vi "BallPlacementEnemyTactic.vi"(8 "error in (no error)":errorcluster, 9 "Robot":refnum<class "Robot.lvclass">, 10 "Game":refnum<class "Game.lvclass">, 11 "BallPlacementEnemyTactic in":refnum<class "BallPlacementEnemyTactic.lvclass">) -> (0 "error out":errorcluster, 2 "Robot out":refnum<class "Robot.lvclass">, 3 "BallPlacementEnemyTactic out":refnum<class "BallPlacementEnemyTactic.lvclass">)   [LabVIEW 2020, in "BallPlacementEnemyTactic.lvclass"]
uses:
  BallPlacementEnemyTactic.lvclass
  Robot_class/Robot.lvclass
  Game_class/Game.lvclass
  Robot_class/tactics.ctl
  Tactic_class/Tactic.lvclass/Tactic.ctl
  Object_class/Object.lvclass/Object.ctl
  Game_class/Game.lvclass/Game.ctl
  Skillbook_class/Skillbook.lvclass/Skillbook.ctl
  Robot_class/Robot.lvclass/Robot.ctl
  <vilib>/Analysis/baseanly.llb/Unit Vector (DBL).vi
  Game_class/Read Referee.vi
  Game_class/Read BallRef.vi
  Object_class/Read x.vi
  Object_class/Read y.vi
  Skillbook_class/Read HaltSkill.vi
  <vilib>/Analysis/coordinate.llb/2D Cartesian Coordinate Rotation (Scalar).vi
  <vilib>/Analysis/baseanly.llb/Real Dot Product.vi
  Robot_class/Write dest_x.vi
  Robot_class/Write dest_y.vi
  Tactic_class/Read Skillbook.vi
  Robot_class/Write tactic.vi
  Ball_class/Ball.lvclass
  Skillbook_class/Skillbook.lvclass
  Referee_class/Referee.lvclass
  HaltSkill_class/HaltSkill.lvclass
  Utilities_class/Utilities.lvclass
  <vilib>/Analysis/NI_AALPro.lvlib
  <vilib>/Analysis/NI_AALBase.lvlib
panel:
  out "x .or. y?":bool
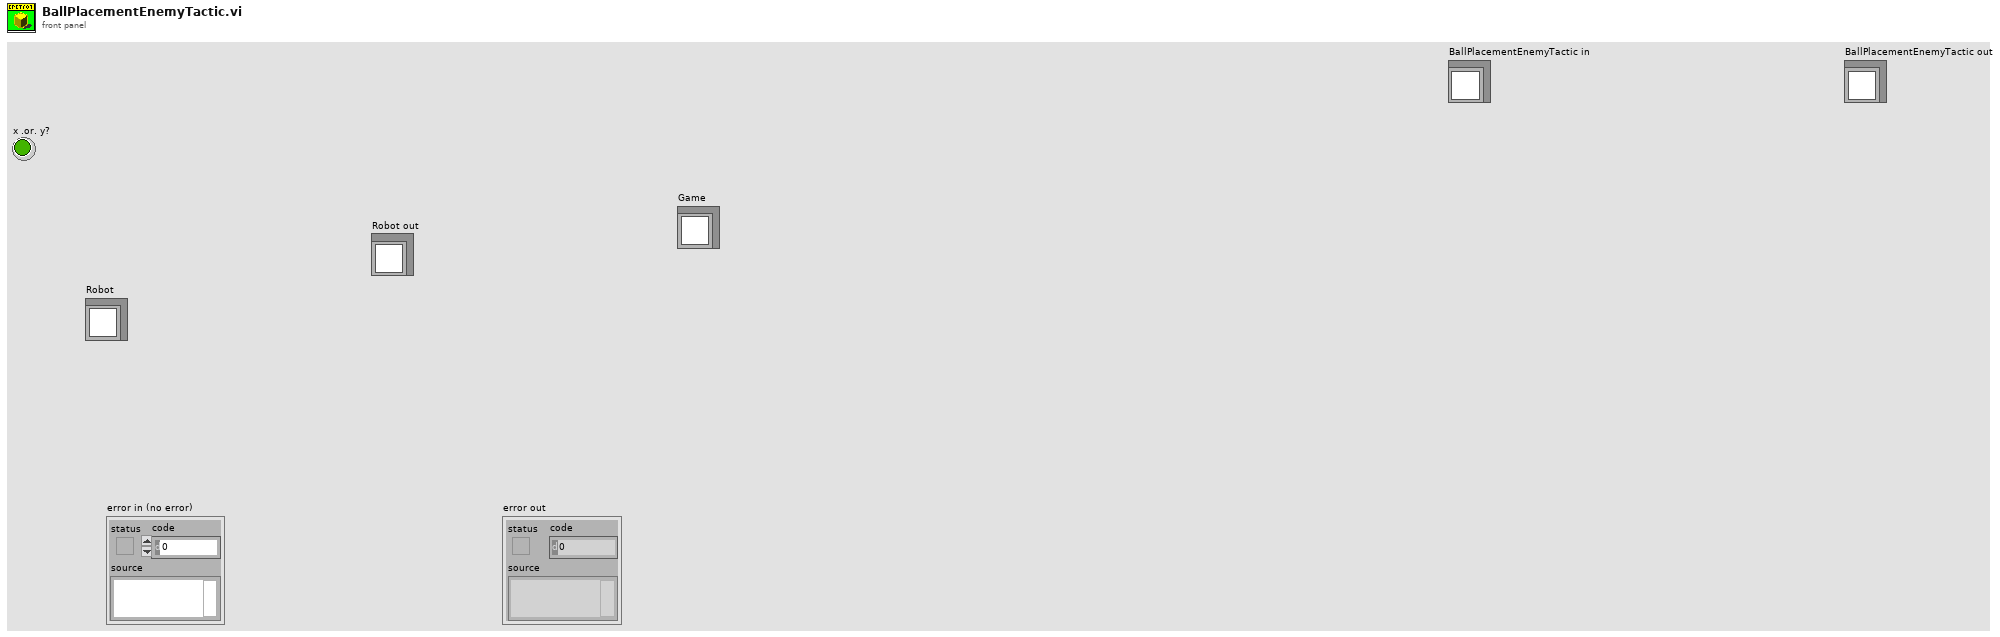
[diagram p1: front panel]
types:
  T1 = typedef "tactics.ctl" = enum16{"5Robots", "BallPlacementEnemy", "ReceivePassInFuturePoint", "Roller", "PrepareRollToPassRollerGoTo", "PrepareRollToPassReceiverGoTo", "WaitRoll", "PositionToRoll", "PenaltyAttacker", "PassObserver", "PenaltyDefense", "TableReceiverTactic", "Test", "DefendGoal", "Marker", "FollowAttacker", "DefendArea", "Shoot", "AttackerAimGoal", "AttackerBallOutOfField", "AttackerBlock", "AttackerStop", "Duelist", "Halt", "ZigZag", "GoTo", "Timeout", "KickToBestRobot", "KickToPassReceiver", "PositionToReceivePass", "WaitPass"}
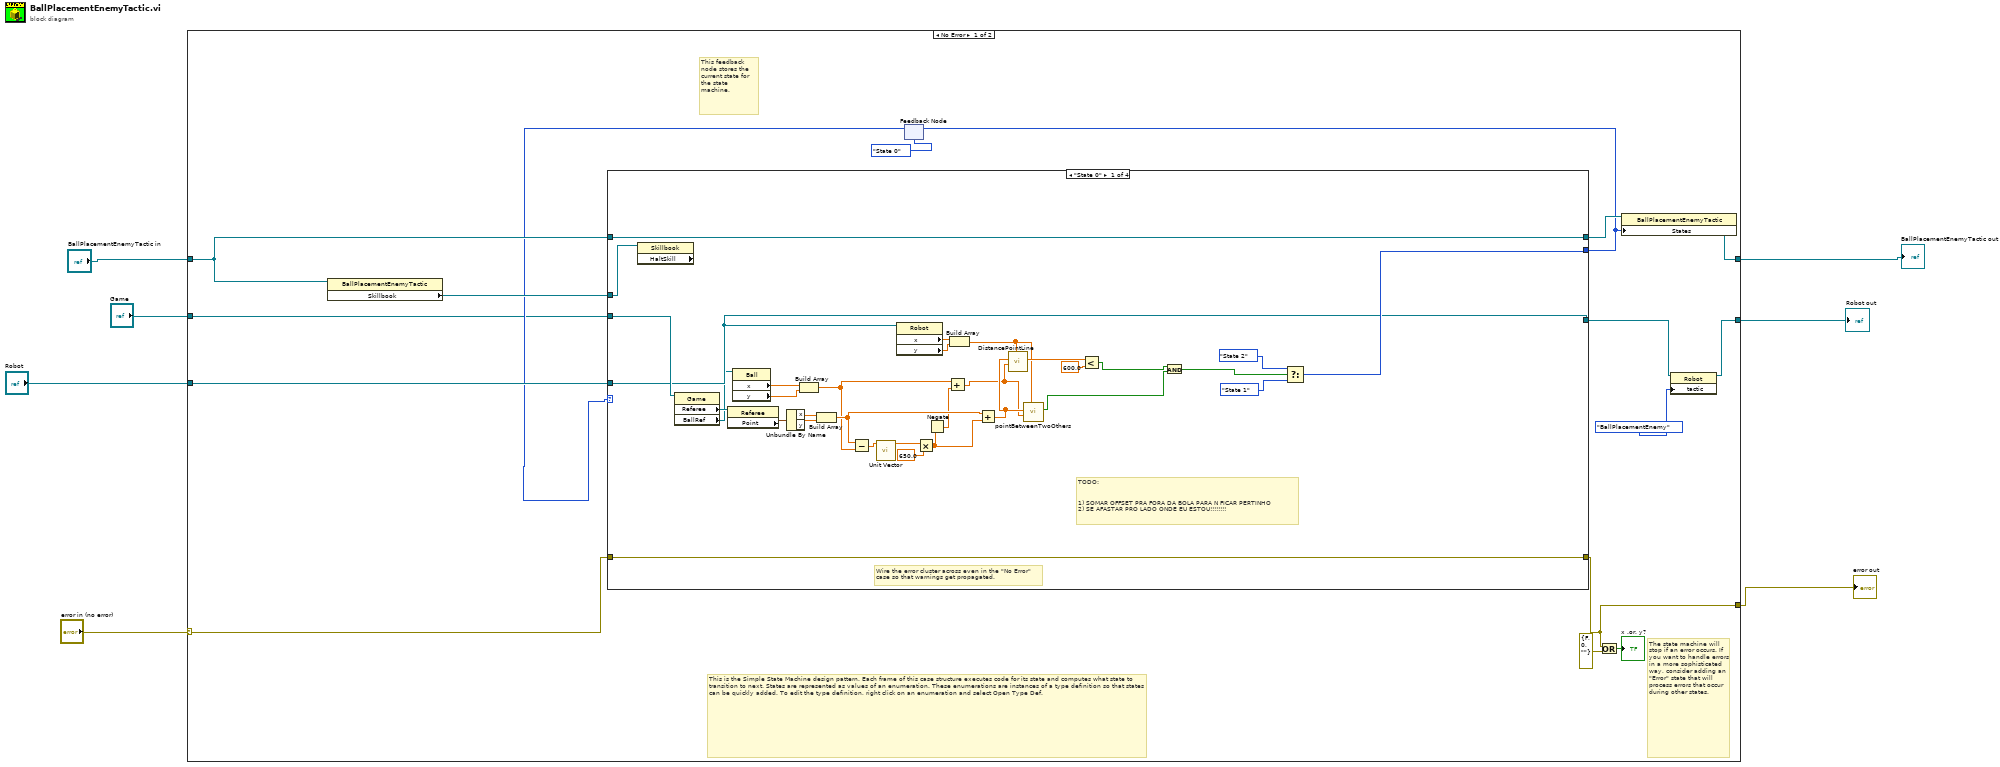
[diagram p0: block diagram]
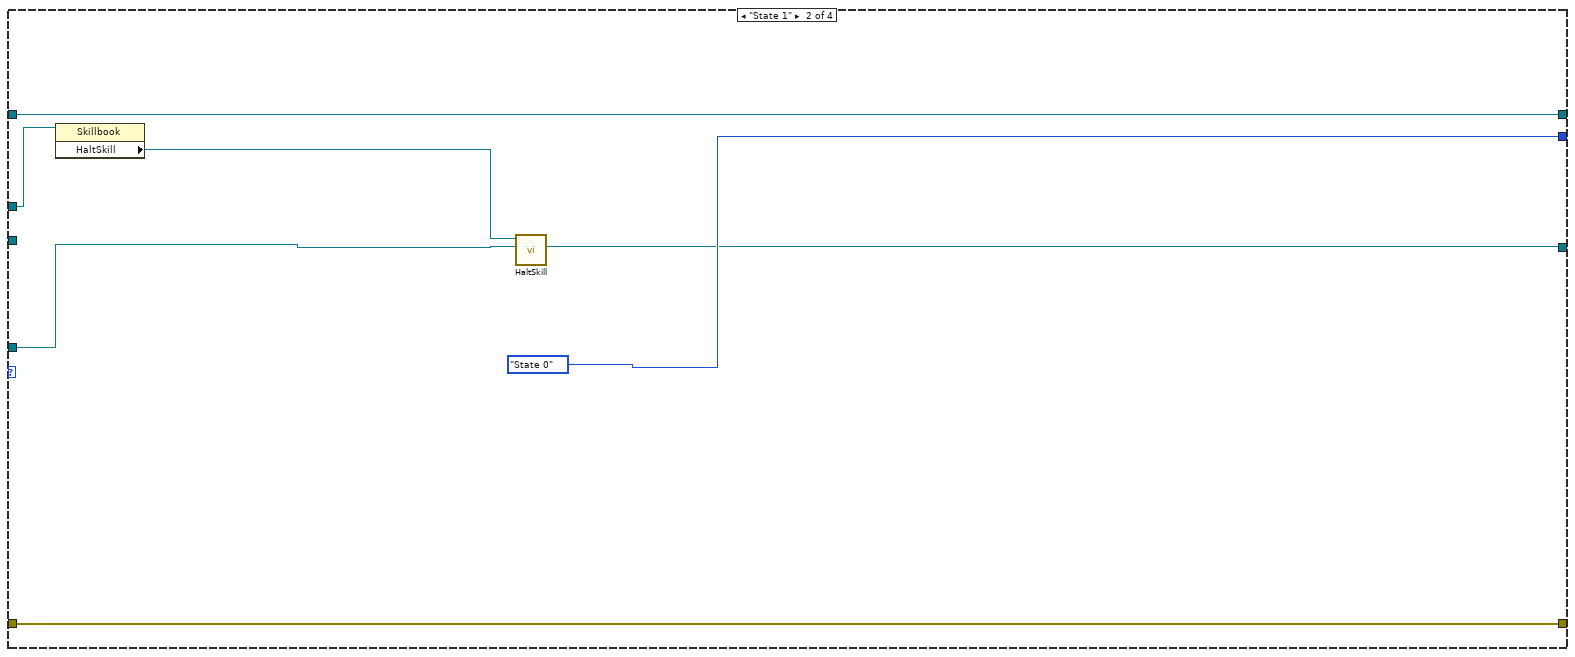
[diagram p2: hidden frame]
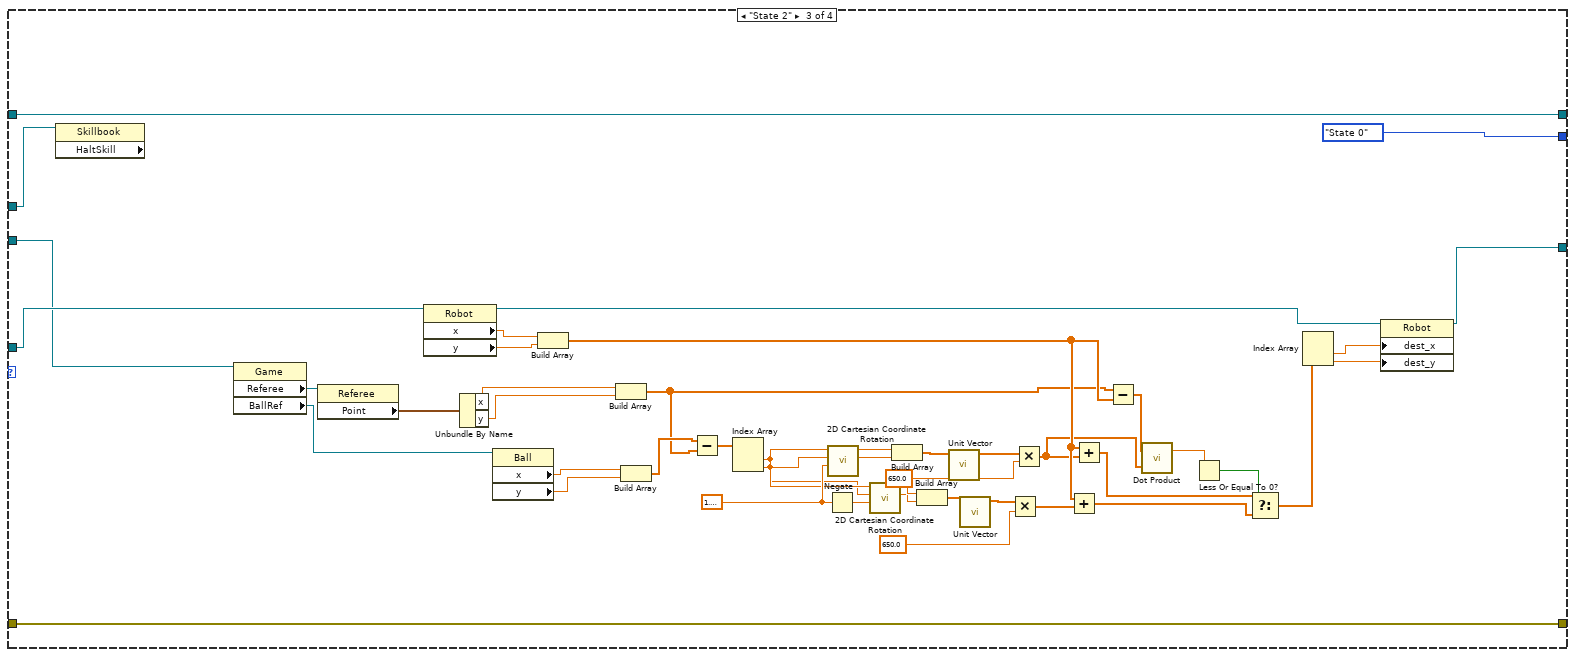
[diagram p3: hidden frame]
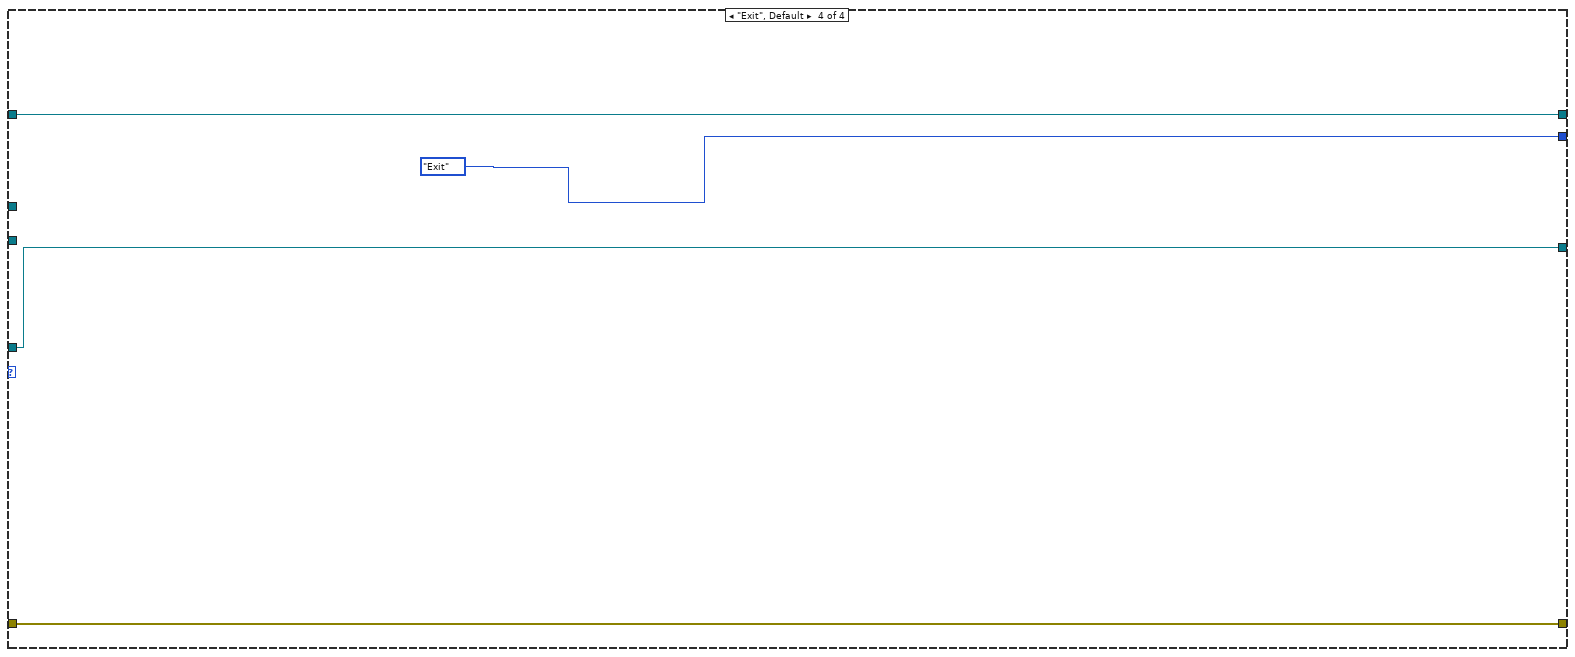
[diagram p4: hidden frame]
diagram:
  n1 = case shown="No Error" "error in (no error)" {
    selector: "error in (no error)" -> [w22 w114]
    tunnel: [w21 w114] -> w6
    tunnel: [w17 w113] -> w1
    tunnel: "BallPlacementEnemyTactic in" -> [w15 w113]
    tunnel: "Robot" -> [w20 w112]
    tunnel: [w12 w112] -> w4
    tunnel: "Game" -> [w8 _]
    frame No Error {
      # "The state machine will stop if an error occurs. If you want to handle errors in a more sophisticated way, consider adding an \"Error\" state that will process errors that occur during other states."
      # "This feedback node stores the current state for the state machine."
      # "This is the Simple State Machine design pattern. Each frame of this case structure executes code for its state and computes what state to transition to next. States are represented as values of an enumeration. These enumerations are instances of a type definition so that states can be quickly added. To edit the type definition, right click on an enumeration and select Open Type Def."
      # "Wire the error cluster across even in the \"No Error\"\ncase so that warnings get propagated."
      n2 = property class="BallPlacementEnemyTactic"(reference=w15) -> ("Skillbook"=w19:refnum<class "Skillbook.lvclass">)  [unwired: 1 in, 2 out]
      n3 = feedback #1(enum16{"State 0", "State 1", "State 2", "Exit"}."State 0" ("States")) -> (w10:enum16{"State 0", "State 1", "State 2", "Exit"})
      n4 = case shown="\"State 0\"" w10 {
        tunnel: w22 -> [w55 w62 w107 w111]
        tunnel: [w55 w62 w107 w111] -> w21
        tunnel: w19 -> [w54 w61 w106 _]
        tunnel: w20 -> [w38 w57 w94 w109]
        tunnel: [w38 w56 w75 w109] -> w13
        tunnel: [w53 w60 w105 w110] -> w18
        tunnel: w15 -> [w53 w60 w105 w110]
        tunnel: w8 -> [w52 _ w93 _]
        tunnel: [w39 enum16{"State 0", "State 1", "State 2", "Exit"}."State 0" ("States") enum16{"State 0", "State 1", "State 2", "Exit"}."State 0" ("States") enum16{"State 0", "State 1", "State 2", "Exit"}."Exit" ("States")] -> w9
        frame "State 0" {
          # "TODO:\n\n\n1) SOMAR OFFSET PRA FORA DA BOLA PARA N FICAR PERTINHO\n2) SE AFASTAR PRO LADO ONDE EU ESTOU!!!!!!!!"
          n5 = property class="Skillbook" props=["HaltSkill"](reference=w54) -> ()  [unwired: 1 in, 3 out]
          n6 = property class="Game"(reference=w52) -> ("Referee"=w51:refnum<class "Referee.lvclass">, "BallRef"=w37:refnum<class "Ball.lvclass">)  [unwired: 1 in, 2 out]
          n7 = property class="Referee"(reference=w51) -> ("Point"=w50:cluster{"x":sgl, "y":sgl})  [unwired: 1 in, 2 out]
          n8 = property class="Ball"(reference=w37) -> ("x"=w47:dbl, "y"=w46:dbl)  [unwired: 1 in, 2 out]
          n9 = Unbundle By Name(w50) -> ("x"=w49:sgl, "y"=w48:sgl)
          n10 = Build Array(w47, w46) -> (w26:dbl[])
          n11 = Build Array(w49, w48) -> (w29:sgl[])
          n12 = Subtract(x=w29, y=w26) -> (x-y=w32:dbl[])
          n13 = call-poly <vilib>:"Unit Vector.vi"("Input Vector"=w32) -> ("Unit Vector"=w31:dbl[])  [unwired: 8 in, 2 out]
          n14 = property class="Robot"(reference=w38) -> ("x"=w45:dbl, "y"=w44:dbl)  [unwired: 1 in, 2 out]
          n15 = Multiply(x=w31, y=650.0) -> (x*y=w28:dbl[])
          n16 = Negate(x=w28) -> (-x=w25:dbl[])
          n17 = Add(x=w26, y=w25) -> (x+y=w24:dbl[])
          n18 = Build Array(w45, w44) -> (w34:dbl[])
          n19 = Add(x=w29, y=w28) -> (x+y=w27:dbl[])
          n20 = call "DistancePointLine.vi"("Q"=w34, "P2"=w24, "P1"=w27) -> ("distance"=w43:dbl)  [unwired: 6 in, 2 out]
          n21 = call "pointBetweenTwoOthers.vi"("Query"=w34, "P2"=w24, "P1"=w27) -> ("queryBetweenP1P2"=w33:bool)  [unwired: 6 in, 2 out]
          n22 = Less?(x=w43, y=600.0) -> (x < y?=w36:bool)
          n23 = And(x=w36, y=w33) -> (x .and. y?=w35:bool)
          n24 = Select(t=enum16{"State 0", "State 1", "State 2", "Exit"}."State 2" ("States"), s=w35, f=enum16{"State 0", "State 1", "State 2", "Exit"}."State 1" ("States")) -> (s? t:f=w39:enum16{"State 0", "State 1", "State 2", "Exit"})
        }
        frame "State 1" {
          n25 = property class="Skillbook"(reference=w61) -> ("HaltSkill"=w58:refnum<class "HaltSkill.lvclass">)  [unwired: 1 in, 2 out]
          n26 = call-dynamic "HaltSkill.vi"("Robot"=w57, "HaltSkill in"=w58) -> ("Robot out"=w56:refnum<class "Robot.lvclass">)  [unwired: 7 in, 2 out]
        }
        frame "State 2" {
          w91 = 1.5707963267948966
          n27 = property class="Skillbook" props=["HaltSkill"](reference=w106) -> ()  [unwired: 1 in, 3 out]
          n28 = property class="Game"(reference=w93) -> ("Referee"=w103:refnum<class "Referee.lvclass">, "BallRef"=w99:refnum<class "Ball.lvclass">)  [unwired: 1 in, 2 out]
          n29 = property class="Referee"(reference=w103) -> ("Point"=w102:cluster{"x":sgl, "y":sgl})  [unwired: 1 in, 2 out]
          n30 = property class="Robot"(reference=w94) -> (reference out=w76:refnum<class "Robot.lvclass">, "x"=w96:dbl, "y"=w95:dbl)  [unwired: 1 in, 1 out]
          n31 = Unbundle By Name(w102) -> ("x"=w101:sgl, "y"=w100:sgl)
          n32 = property class="Ball"(reference=w99) -> ("x"=w98:dbl, "y"=w97:dbl)  [unwired: 1 in, 2 out]
          n33 = Build Array(w96, w95) -> (w73:dbl[])
          n34 = Build Array(w101, w100) -> (w72:sgl[])
          n35 = Build Array(w98, w97) -> (w74:dbl[])
          n36 = Subtract(x=w74, y=w72) -> (x-y=w78:dbl[])
          n37 = Index Array(array=w78) -> (element #1=w90:dbl, element #2=w89:dbl)  [unwired: 2 in]
          n38 = Negate(x=w91) -> (-x=w92:dbl)
          n39 = call-poly <vilib>:"2D Cartesian Coordinate Rotation.vi"("theta"=w91, "y"=w89, "x"=w90) -> ("y out"=w87:dbl, "x out"=w88:dbl)  [unwired: 6 in, 1 out]
          n40 = call-poly <vilib>:"2D Cartesian Coordinate Rotation.vi"("theta"=w92, "y"=w89, "x"=w90) -> ("y out"=w85:dbl, "x out"=w86:dbl)  [unwired: 6 in, 1 out]
          n41 = Build Array(w88, w87) -> (w84:dbl[])
          n42 = Build Array(w86, w85) -> (w83:dbl[])
          n43 = call-poly <vilib>:"Unit Vector.vi"("Input Vector"=w84) -> ("Unit Vector"=w82:dbl[])  [unwired: 8 in, 2 out]
          n44 = call-poly <vilib>:"Unit Vector.vi"("Input Vector"=w83) -> ("Unit Vector"=w81:dbl[])  [unwired: 8 in, 2 out]
          n45 = Multiply(x=w81, y=650.0) -> (x*y=w77:dbl[])
          n46 = Multiply(x=w82, y=650.0) -> (x*y=w64:dbl[])
          n47 = Add(x=w73, y=w77) -> (x+y=w68:dbl[])
          n48 = Add(x=w73, y=w64) -> (x+y=w63:dbl[])
          n49 = Subtract(x=w72, y=w73) -> (x-y=w71:dbl[])
          n50 = call-poly <vilib>:"Dot Product.vi"("Y Vector"=w64, "X Vector"=w71) -> ("X * Y"=w70:dbl)  [unwired: 1 out]
          n51 = Less Or Equal To 0?(x=w70) -> (x <= 0?=w69:bool)
          n52 = Select(t=w63, s=w69, f=w68) -> (s? t:f=w67:dbl[])
          n53 = Index Array(array=w67) -> (element #1=w66:dbl, element #2=w65:dbl)  [unwired: 2 in]
          n54 = property class="Robot"(reference=w76, "dest_x"=w66, "dest_y"=w65) -> (reference out=w75:refnum<class "Robot.lvclass">)  [unwired: 1 in, 1 out]
        }
        frame "Exit", Default {
        }
      }
      n55 = feedback-in #1(w9) -> ()
      n56 = Or(x=w21, y=errorcluster {"status"=FALSE, "code"=0, "source"=""}) -> (x .or. y?=→"x .or. y?":bool)
      n57 = property class="BallPlacementEnemyTactic"(reference=w18, "States"=w9) -> (reference out=w17:refnum<class "BallPlacementEnemyTactic.lvclass">)  [unwired: 1 in, 1 out]
      n58 = property class="Robot"(reference=w13, "tactic"=tactics."BallPlacementEnemy") -> (reference out=w12:refnum<class "Robot.lvclass">)  [unwired: 1 in, 1 out]
    }
    frame Error {
    }
  }
  "BallPlacementEnemyTactic out" <- w1
  "error out" <- w6
  "Robot out" <- w4
